vi "#148_MAV_MSG_AUTOPILOT_VERSION_DECODE.vi"(11 "mavlink_payload":u8[](array[numeric])) -> (3 "AUTOPILOT_VERSION":T1)   [LabVIEW 2023]
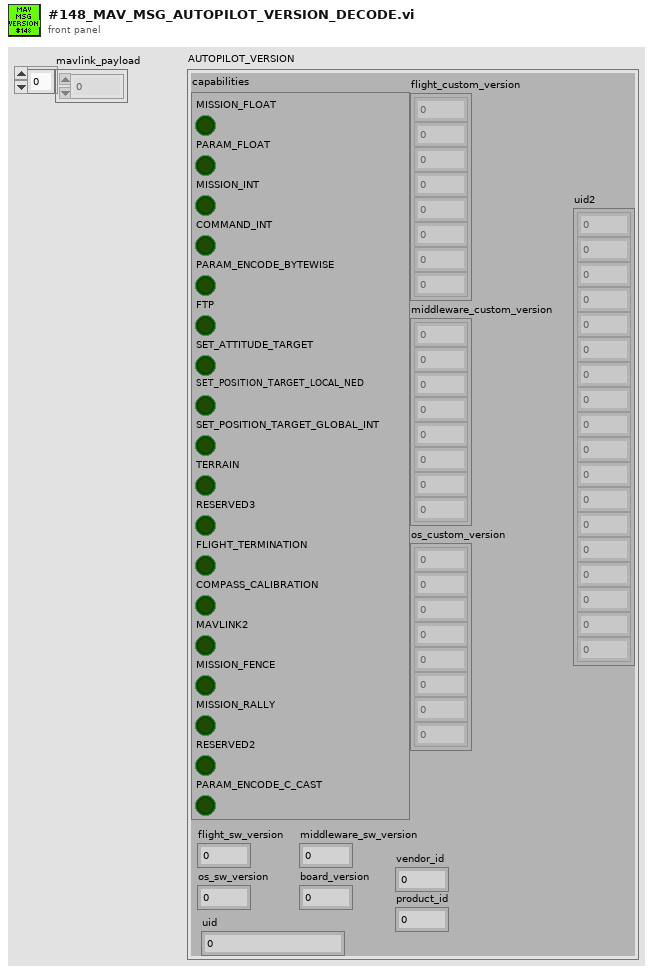
[diagram p1: front panel]
types:
  T1 = cluster{"flight_sw_version":u32, "middleware_sw_version":u32, "os_sw_version":u32, "board_version":u32, "capabilities":cluster{"MISSION_FLOAT":bool, "PARAM_FLOAT":bool, "MISSION_INT":bool, "COMMAND_INT":bool, "PARAM_ENCODE_BYTEWISE":bool, "FTP":bool, "SET_ATTITUDE_TARGET":bool, "SET_POSITION_TARGET_LOCAL_NED":bool, "SET_POSITION_TARGET_GLOBAL_INT":bool, "TERRAIN":bool, "RESERVED3":bool, "FLIGHT_TERMINATION":bool, "COMPASS_CALIBRATION":bool, "MAVLINK2":bool, "MISSION_FENCE":bool, "MISSION_RALLY":bool, "RESERVED2":bool, "PARAM_ENCODE_C_CAST":bool}, "flight_custom_version":u8[], "middleware_custom_version":u8[], "os_custom_version":u8[], "vendor_id":u16, "product_id":u16, "uid":u64, "uid2":u8[]}
  T2 = cluster{"Boolean array[0]":bool, "Boolean array[1]":bool, "Boolean array[2]":bool, "Boolean array[3]":bool, "Boolean array[4]":bool, "Boolean array[5]":bool, "Boolean array[6]":bool, "Boolean array[7]":bool, "Boolean array[8]":bool, "Boolean array[9]":bool, "Boolean array[10]":bool, "Boolean array[11]":bool, "Boolean array[12]":bool, "Boolean array[13]":bool, "Boolean array[14]":bool, "Boolean array[15]":bool, "Boolean array[16]":bool, "Boolean array[17]":bool}
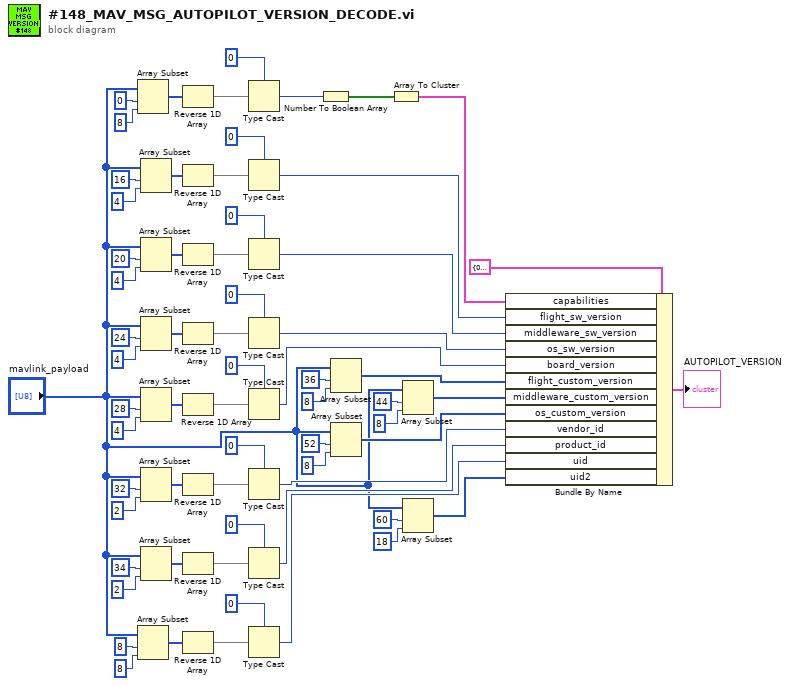
[diagram p0: block diagram]
diagram:
  n1 = Array Subset(array="mavlink_payload", index=0 ("Index"), length=8) -> (w62:u8[])
  n2 = Array Subset(array="mavlink_payload", index=8 ("Index"), length=8) -> (w9:u8[])
  n3 = Array Subset(array="mavlink_payload", index=16 ("Index"), length=4) -> (w54:u8[])
  n4 = Array Subset(array="mavlink_payload", index=20 ("Index"), length=4) -> (w48:u8[])
  n5 = Array Subset(array="mavlink_payload", index=24 ("Index"), length=4) -> (w42:u8[])
  n6 = Array Subset(array="mavlink_payload", index=28 ("Index"), length=4) -> (w36:u8[])
  n7 = Array Subset(array="mavlink_payload", index=32 ("Index"), length=2) -> (w21:u8[])
  n8 = Array Subset(array="mavlink_payload", index=34 ("Index"), length=2) -> (w15:u8[])
  n9 = Reverse 1D Array(array=w62) -> (reversed array=w61:u8[])
  n10 = Reverse 1D Array(array=w54) -> (reversed array=w53:u8[])
  n11 = Reverse 1D Array(array=w48) -> (reversed array=w47:u8[])
  n12 = Reverse 1D Array(array=w42) -> (reversed array=w41:u8[])
  n13 = Reverse 1D Array(array=w36) -> (reversed array=w35:u8[])
  n14 = Reverse 1D Array(array=w21) -> (reversed array=w20:u8[])
  n15 = Reverse 1D Array(array=w15) -> (reversed array=w14:u8[])
  n16 = Reverse 1D Array(array=w9) -> (reversed array=w8:u8[])
  n17 = Type Cast(type=u64 0 ("Index"), x=w61) -> (*(type *) &x=w58:u64)
  n18 = Type Cast(type=u32 0 ("Index"), x=w53) -> (*(type *) &x=w50:u32)
  n19 = Type Cast(type=u32 0 ("Index"), x=w47) -> (*(type *) &x=w44:u32)
  n20 = Type Cast(type=u32 0 ("Index"), x=w41) -> (*(type *) &x=w38:u32)
  n21 = Type Cast(type=u32 0 ("Index"), x=w35) -> (*(type *) &x=w32:u32)
  n22 = Type Cast(type=u16 0 ("Index"), x=w20) -> (*(type *) &x=w17:u16)
  n23 = Type Cast(type=u16 0 ("Index"), x=w14) -> (*(type *) &x=w11:u16)
  n24 = Type Cast(type=u64 0 ("Index"), x=w8) -> (*(type *) &x=w5:u64)
  n25 = Number To Boolean Array(number=w58) -> (Boolean array=w57:bool[])
  n26 = Array Subset(array="mavlink_payload", index=36 ("Index"), length=8) -> (w29:u8[])
  n27 = Array Subset(array="mavlink_payload", index=52 ("Index"), length=8) -> (w23:u8[])
  n28 = Array To Cluster(array=w57) -> (cluster=w56:T2)
  n29 = Array Subset(array="mavlink_payload", index=44 ("Index"), length=8) -> (w26:u8[])
  n30 = Array Subset(array="mavlink_payload", index=60 ("Index"), length=18) -> (w1:u8[])
  n31 = Bundle By Name(cluster=T1 {"flight_sw_version"=0, "middleware_sw_version"=0, "os_sw_version"=0, "board_version"=0, "capabilities"={"MISSION_FLOAT"=FALSE, "PARAM_FLOAT"=FALSE, "MISSION_INT"=FALSE, "COMMAND_INT"=FALSE, "PARAM_ENCODE_BYTEWISE"=FALSE, "FTP"=FALSE, "SET_ATTITUDE_TARGET"=FALSE, "SET_POSITION_TARGET_LOCAL_NED"=FALSE, "SET_POSITION_TARGET_GLOBAL_INT"=FALSE, "TERRAIN"=FALSE, "RESERVED3"=FALSE, "FLIGHT_TERMINATION"=FALSE, "COMPASS_CALIBRATION"=FALSE, "MAVLINK2"=FALSE, "MISSION_FENCE"=FALSE, "MISSION_RALLY"=FALSE, "RESERVED2"=FALSE, "PARAM_ENCODE_C_CAST"=FALSE}, "flight_custom_version"=[0, 0, 0, 0, 0, 0, 0, 0], "middleware_custom_version"=[0, 0, 0, 0, 0, 0, 0, 0], "os_custom_version"=[0, 0, 0, 0, 0, 0, 0, 0], "vendor_id"=0, "product_id"=0, "uid"=0, "uid2"=[0, 0, 0, 0, 0, 0, 0, 0, 0, 0, 0, 0, 0, 0, 0, 0, 0, 0]} ("AUTOPILOT_VERSION"), "capabilities"=w56, "flight_sw_version"=w50, "middleware_sw_version"=w44, "os_sw_version"=w38, "board_version"=w32, "flight_custom_version"=w29, "middleware_custom_version"=w26, "os_custom_version"=w23, "vendor_id"=w17, "product_id"=w11, "uid"=w5, "uid2"=w1) -> (→"AUTOPILOT_VERSION":T1)
